vi "Facade.vi"(0 "Data In":T6, 2 "Display State In":T3, 3 "Container State":T5) -> (6 "Data Out":T6, 7 "Display State Out":T3, 8 "Action":T2)   [LabVIEW 2020, in "TTLController.xctl"]
uses:
  TTLController.xctl
  Data.ctl
  Control Classes/Base Class/TTLController.lvclass
  <vilib>/_xctls/Container State.ctl
  State.ctl
  Device Classes/Base Class/TTLControlledDevice.lvclass
  Events.ctl
  Event Type.ctl
  Height Change.vi
  <vilib>/_xctls/Action.ctl
  epl-vi-lib/Utility VIs/Buttons/KCheckmarkBoolean 2.ctl
  Trigger XControl/Trigger.xctl
  Control Classes/Base Class/TTLController.lvclass/TTLController.ctl
  Device Classes/Base Class/TTLControlledDevice.lvclass/TTLControlledDevice.ctl
  Control Classes/Base Class/Read Start .vi
  Control Classes/Base Class/Read Stop .vi
  Control Classes/Base Class/Read Active.vi
  Control Classes/Base Class/Read IPI.vi
  Control Classes/Base Class/Read Width (ms).vi
  Device Classes/Base Class/Read Name.vi
  Control Classes/Base Class/Write Start .vi
  Control Classes/Base Class/Write Active.vi
  Control Classes/Base Class/Write IPI.vi
  Control Classes/Base Class/Write Width (ms).vi
  Control Classes/Base Class/Write Stop .vi
  <vilib>/_xctls/XControlSupport.lvlib
panel:
  in  "IPI (ms)":string
  in  "Mode":enum16{"Constant", "Pulsed"}(ring)
  in  "Width":dbl caption="Width (ms)"
  in  "Stop":cluster{"When":string, "Expr":string}(xcontrol)
  in  "Start":cluster{"When":string, "Expr":string}(xcontrol)
  out "Icon":picture
  in  "Active":T1
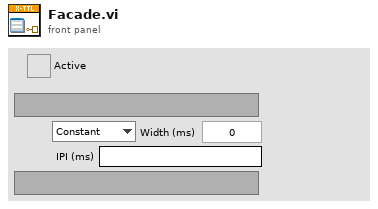
[diagram p1: front panel]
types:
  T1 = typedef "KCheckmarkBoolean 2.ctl" = bool
  T2 = typedef "XControlSupport.lvlib/Action.ctl" = cluster{"Data Changed?":bool, "State Changed?":bool, "Action Name":string}
  T3 = typedef "TTLController.xctl/State.ctl" = cluster{"Active":bool, "Device":refnum<class "TTLControlledDevice.lvclass">, "Events":T4, "Height":i32}
  T4 = typedef "TTLController.xctl/Events.ctl" = cluster{"Generic":refnum<user-event>, "Height":refnum<user-event>}
  T5 = typedef "XControlSupport.lvlib/Container State.ctl" = cluster{"Indicator?":bool, "Run Mode?":bool, " Refnum":refnum<vi>}
  T6 = typedef "TTLController.xctl/Data.ctl" = refnum<class "TTLController.lvclass">
  T7 = typedef "TTLController.lvclass/Trigger.ctl" = cluster{"When":string, "Expr":string}
  T8 = typedef "LVPoint32TypeDef.ctl" = cluster{"Horizontal":i32, "Vertical":i32}
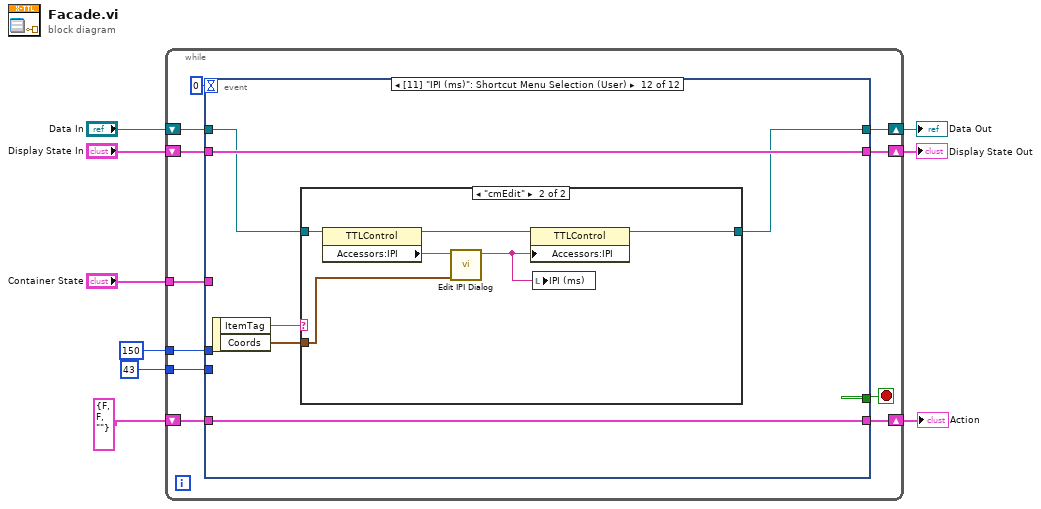
[diagram p0: block diagram]
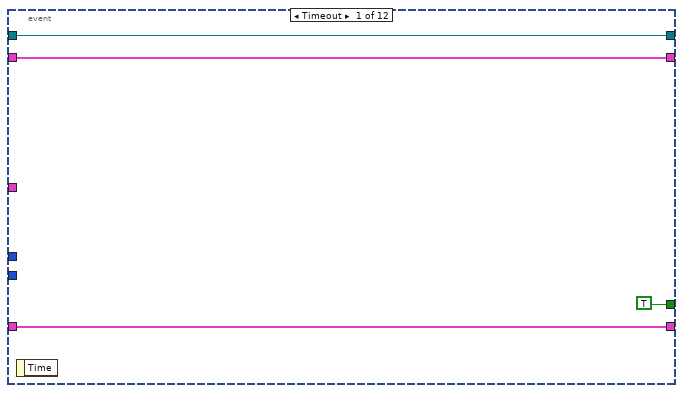
[diagram p2: hidden frame]
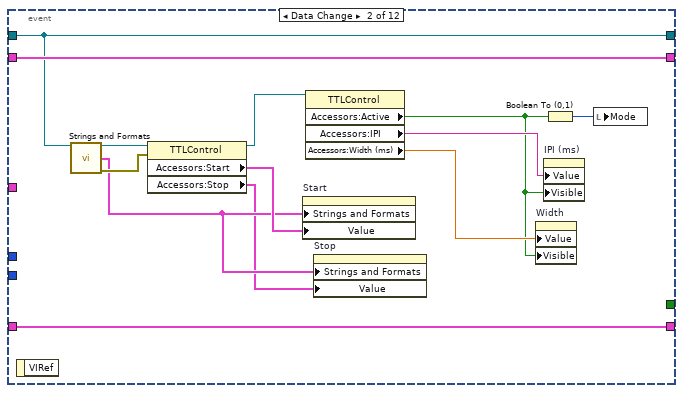
[diagram p3: hidden frame]
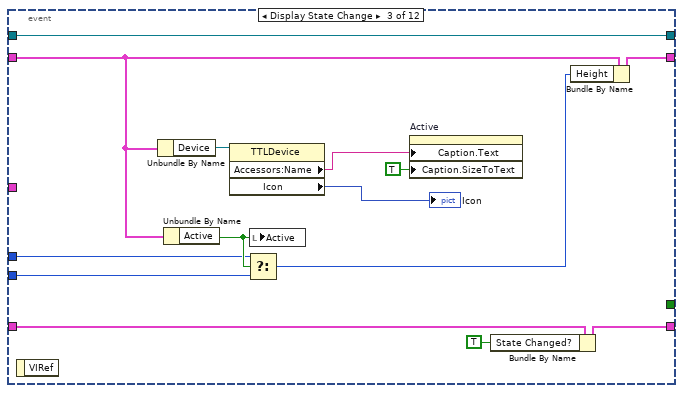
[diagram p4: hidden frame]
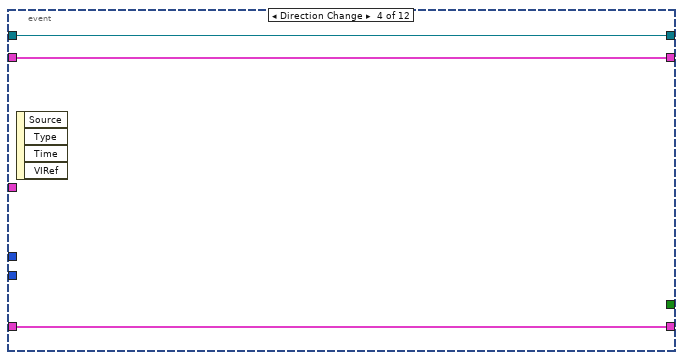
[diagram p5: hidden frame]
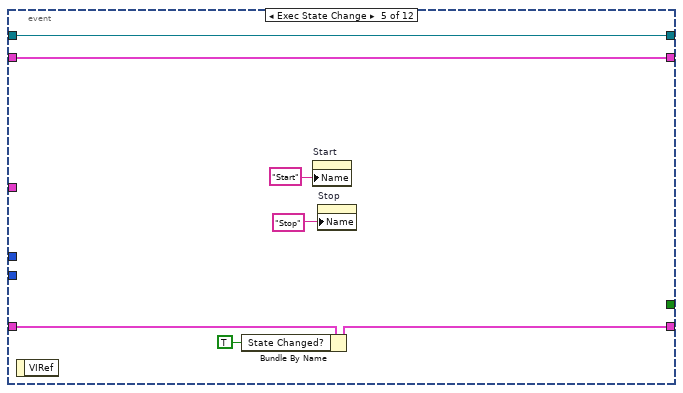
[diagram p6: hidden frame]
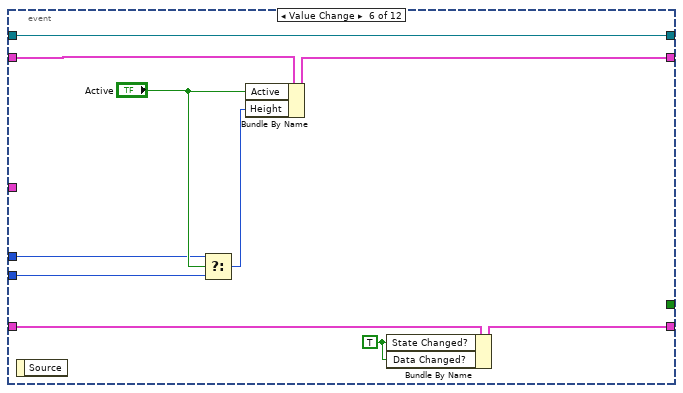
[diagram p7: hidden frame]
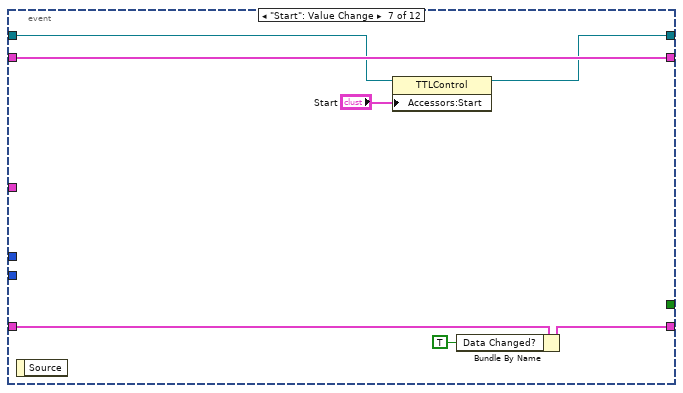
[diagram p8: hidden frame]
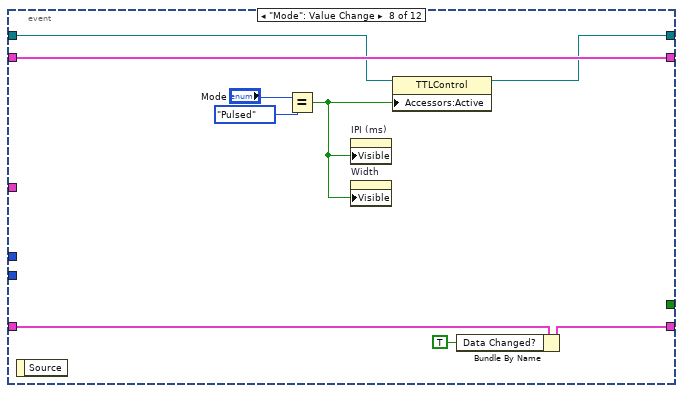
[diagram p9: hidden frame]
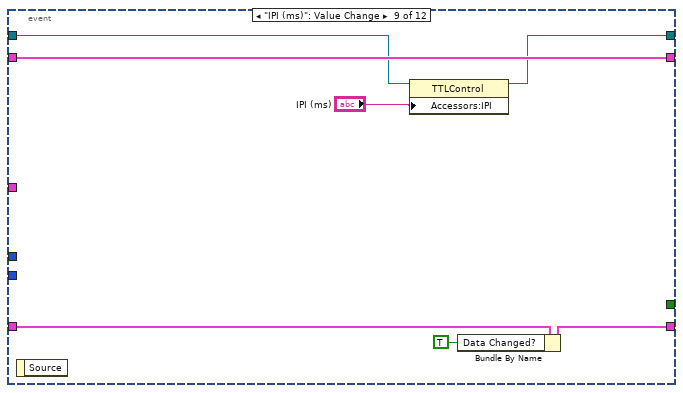
[diagram p10: hidden frame]
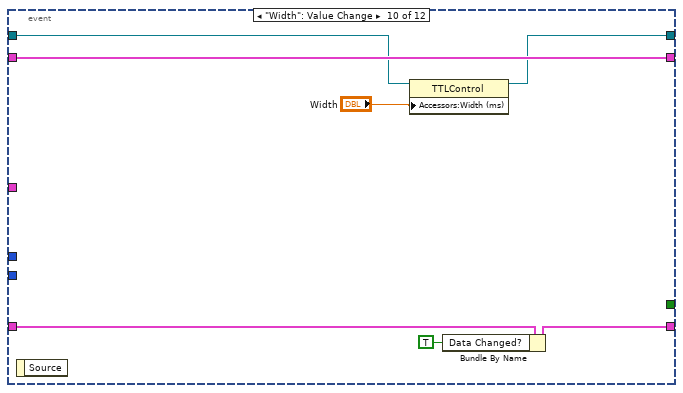
[diagram p11: hidden frame]
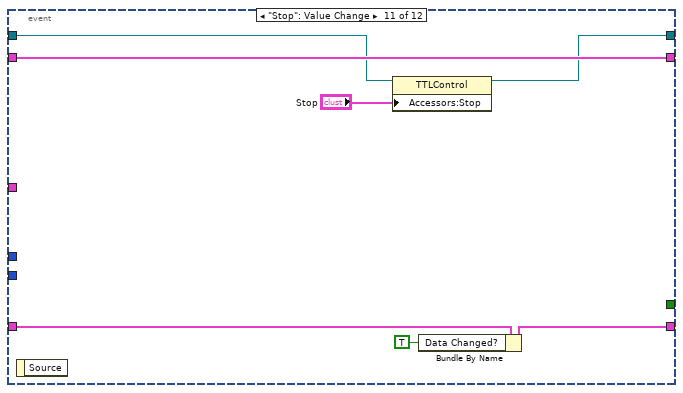
[diagram p12: hidden frame]
diagram:
  n1 = while {
    shift-right: [w19] -> w6
    shift-left: "Display State In" -> [w20]
    tunnel: "Container State" -> [w16]
    shift-right: [w14] -> w9
    shift-left: "Data In" -> [w15]
    shift-right: [w12] -> w4
    shift-left: T2 {"Data Changed?"=FALSE, "State Changed?"=FALSE, "Action Name"=""} ("Action") -> [w13]
    tunnel: 150 -> [w11]
    tunnel: 43 -> [w10]
    stop <- w18 stop-if-true
    n2 = event shown="[11] \"IPI (ms)\": Shortcut Menu Selection (User)" {
      selector: _ -> [_ _ _ _ _ _ _ _ _ _ _ _]
      dyn-events: _ -> [_ _ _ _ _ _ _ _ _ _ _ _]
      timeout: 0 -> [_ _ _ _ _ _ _ _ _ _ _ _]
      tunnel: w20 -> [w22 w37 w46 w54 w57 w64 w78 w87 w94 w101 w108 w114]
      tunnel: [w22 w37 w40 w54 w57 w65 w78 w87 w94 w101 w108 w114] -> w19
      tunnel: [TRUE _ _ _ _ _ _ _ _ _ _ _] -> w18
      tunnel: w16 -> [_ _ _ _ _ _ _ _ _ _ _ _]
      tunnel: w15 -> [w21 w35 w51 w53 w61 w71 w77 w86 w93 w100 w107 w111]
      tunnel: [w21 w35 w51 w53 w61 w71 w75 w84 w91 w98 w105 w110] -> w14
      tunnel: [w23 w36 w42 w52 w56 w66 w73 w83 w90 w96 w103 w113] -> w12
      tunnel: w13 -> [w23 w36 w50 w52 w60 w70 w76 w85 w92 w99 w106 w113]
      tunnel: w11 -> [_ _ w44 _ _ w68 _ _ _ _ _ _]
      tunnel: w10 -> [_ _ w43 _ _ w67 _ _ _ _ _ _]
      event Timeout {
        n3 = event-data() -> ()  [unwired: 1 in, 1 out]
      }
      event Data Change {
        n4 = event-data() -> ()  [unwired: 1 in, 1 out]
        n5 = call-dynamic "Strings and Formats.vi"("TTLControl in"=w35) -> ("TTLControl out"=w34:T6, "Strings[] and Formats[]"=w31:cluster{"Strings":string[], "Formats":string[]}, "error out"=w33:errorcluster)  [unwired: 12 in]
        n6 = property class="TTLControl"(reference=w34, error in=w33) -> (reference out=w29:T6, "Accessors:Start "=w32:T7, "Accessors:Stop "=w30:T7)  [unwired: 1 out]
        n7 = property on="Start" class="Trigger (strict)"("Strings and Formats"=w31, "Value"=w32) -> ()  [unwired: 2 in, 2 out]
        n8 = property class="TTLControl"(reference=w29) -> ("Accessors:Active"=w25:bool, "Accessors:IPI"=w26:string, "Accessors:Width (ms)"=w27:dbl)  [unwired: 1 in, 2 out]
        n9 = property on="Stop" class="Trigger (strict)"("Strings and Formats"=w31, "Value"=w30) -> ()  [unwired: 2 in, 2 out]
        n10 = property on="Width" class="DigNum (strict)"("Value"=w27, "Visible"=w25) -> ()  [unwired: 2 in, 2 out]
        n11 = property on="IPI (ms)" class="Str"("Value"=w26, "Visible"=w25) -> ()  [unwired: 2 in, 2 out]
        n12 = Boolean To (0,1)(Boolean=w25) -> (0, 1=w28:i16)
        n13 = local write "Mode"(w28) -> ()
      }
      event Display State Change {
        n14 = event-data() -> ()  [unwired: 1 in, 1 out]
        n15 = Unbundle By Name(w46) -> ("Device"=w49:refnum<class "TTLControlledDevice.lvclass">)
        n16 = Unbundle By Name(w46) -> ("Active"=w45:bool)
        n17 = property class="TTLDevice"(reference=w49) -> ("Accessors:Name"=w48:string, "Icon"=→"Icon":picture)  [unwired: 1 in, 2 out]
        n18 = Select(t=w44, s=w45, f=w43) -> (s? t:f=w39:i32)
        n19 = local write "Active"(w45) -> ()
        n20 = property on="Active" class="Bool (strict)"("Caption.Text"=w48, "Caption.SizeToText"=TRUE ("Caption.Size to Text?")) -> ()  [unwired: 2 in, 2 out]
        n21 = Bundle By Name(cluster=w50, "State Changed?"=TRUE) -> (w42:T2)
        n22 = Bundle By Name(cluster=w46, "Height"=w39) -> (w40:T3)
      }
      event Direction Change {
        n23 = event-data() -> ()  [unwired: 1 in, 4 out]
      }
      event Exec State Change {
        n24 = event-data() -> ()  [unwired: 1 in, 1 out]
        n25 = Bundle By Name(cluster=w60, "State Changed?"=TRUE) -> (w56:T2)
        n26 = property on="Start" class="Trigger (strict)"("Name"="Start") -> ()  [unwired: 2 in, 2 out]
        n27 = property on="Stop" class="Trigger (strict)"("Name"="Stop") -> ()  [unwired: 2 in, 2 out]
      }
      event Value Change {
        w62 = TRUE ("State Changed?")
        n28 = event-data() -> ()  [unwired: 1 in, 1 out]
        n29 = Select(t=w68, s="Active", f=w67) -> (s? t:f=w63:i32)
        n30 = Bundle By Name(cluster=w64, "Active"="Active", "Height"=w63) -> (w65:T3)
        n31 = Bundle By Name(cluster=w70, "State Changed?"=w62, "Data Changed?"=w62) -> (w66:T2)
      }
      event "Start": Value Change {
        n32 = event-data() -> ()  [unwired: 1 in, 1 out]
        n33 = property class="TTLControl"(reference=w77, "Accessors:Start "="Start") -> (reference out=w75:T6)  [unwired: 1 in, 1 out]
        n34 = Bundle By Name(cluster=w76, "Data Changed?"=TRUE) -> (w73:T2)
      }
      event "Mode": Value Change {
        n35 = event-data() -> ()  [unwired: 1 in, 1 out]
        n36 = Equal?(x="Mode", y=enum16{"Constant", "Pulsed"}."Pulsed") -> (x = y?=w79:bool)
        n37 = property on="IPI (ms)" class="Str"("Visible"=w79) -> ()  [unwired: 2 in, 2 out]
        n38 = property on="Width" class="DigNum (strict)"("Visible"=w79) -> ()  [unwired: 2 in, 2 out]
        n39 = property class="TTLControl"(reference=w86, "Accessors:Active"=w79) -> (reference out=w84:T6)  [unwired: 1 in, 1 out]
        n40 = Bundle By Name(cluster=w85, "Data Changed?"=TRUE) -> (w83:T2)
      }
      event "IPI (ms)": Value Change {
        n41 = event-data() -> ()  [unwired: 1 in, 1 out]
        n42 = property class="TTLControl"(reference=w93, "Accessors:IPI"="IPI (ms)") -> (reference out=w91:T6)  [unwired: 1 in, 1 out]
        n43 = Bundle By Name(cluster=w92, "Data Changed?"=TRUE) -> (w90:T2)
      }
      event "Width": Value Change {
        n44 = event-data() -> ()  [unwired: 1 in, 1 out]
        n45 = property class="TTLControl"(reference=w100, "Accessors:Width (ms)"="Width") -> (reference out=w98:T6)  [unwired: 1 in, 1 out]
        n46 = Bundle By Name(cluster=w99, "Data Changed?"=TRUE) -> (w96:T2)
      }
      event "Stop": Value Change {
        n47 = event-data() -> ()  [unwired: 1 in, 1 out]
        n48 = property class="TTLControl"(reference=w107, "Accessors:Stop "="Stop") -> (reference out=w105:T6)  [unwired: 1 in, 1 out]
        n49 = Bundle By Name(cluster=w106, "Data Changed?"=TRUE) -> (w103:T2)
      }
      event "IPI (ms)": Shortcut Menu Selection (User) {
        n50 = event-data() -> ("ItemTag"=w112:string, "Coords"=w109:T8)  [unwired: 1 in]
        n51 = case shown="\"cmEdit\"" w112 {
          tunnel: w111 -> [w115 w121]
          tunnel: [w115 w118] -> w110
          tunnel: w109 -> [_ w117]
          frame "", Default {
          }
          frame "cmEdit" {
            n52 = property class="TTLControl"(reference=w121) -> (reference out=w119:T6, "Accessors:IPI"=w120:string)  [unwired: 1 in, 1 out]
            n53 = call "Edit IPI Dialog.vi"("Coords"=w117, "Expr In"=w120) -> ("Expr Out"=w116:string)  [unwired: 9 in]
            n54 = property class="TTLControl"(reference=w119, "Accessors:IPI"=w116) -> (reference out=w118:T6)  [unwired: 1 in, 1 out]
            n55 = local write "IPI (ms)"(w116) -> ()
          }
        }
      }
    }
  }
  "Display State Out" <- w6
  "Data Out" <- w9
  "Action" <- w4
